vi "TimerHelper.vi"() -> ()   [LabVIEW 2016]
panel:
  in  "Stop":bool
  in  "Pause/Resume":bool
  in  "Start":bool
  in  "Reset":bool
  out "Clock":dbl format="%#_6f"
  # "STOPWATCH"
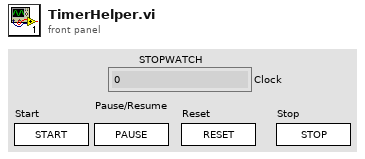
[diagram p1: front panel]
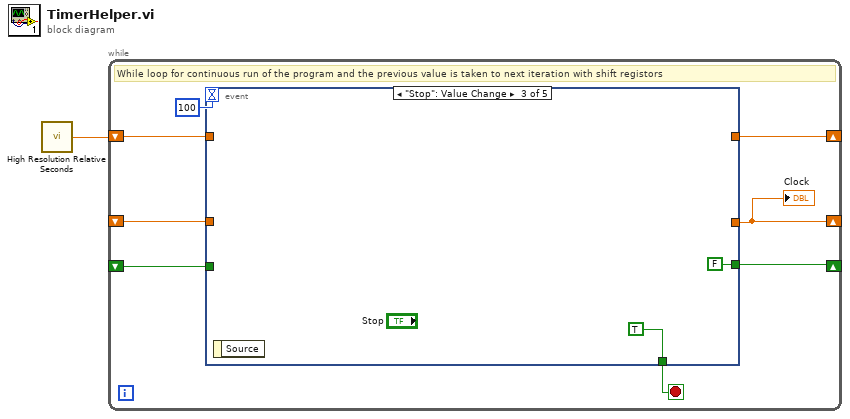
[diagram p0: block diagram]
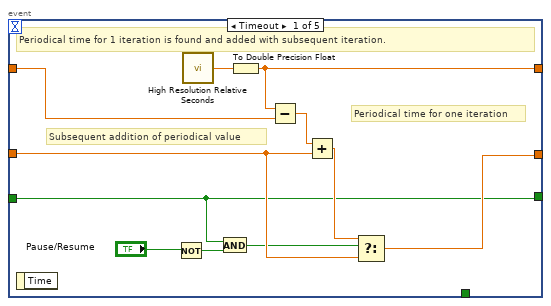
[diagram p2: hidden frame]
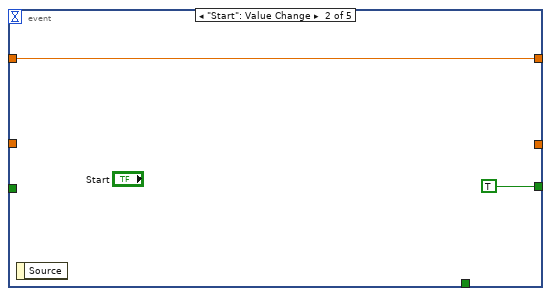
[diagram p3: hidden frame]
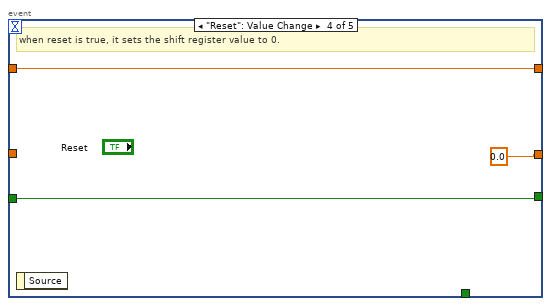
[diagram p4: hidden frame]
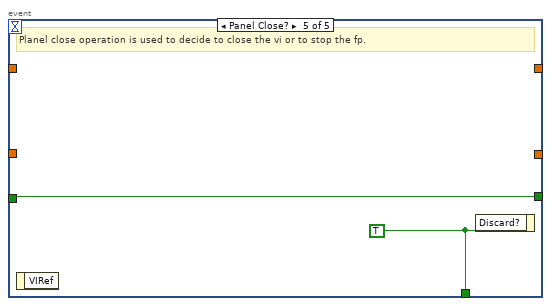
[diagram p5: hidden frame]
diagram:
  n1 = call <vilib>:"High Resolution Relative Seconds.vi"() -> ("relative seconds"=w1:dbl)
  n2 = while {
    shift-right: [w5] -> _
    shift-left: _ -> [w9]
    shift-right: [w8] -> _
    shift-left: w1 -> [w7]
    shift-right: [w3] -> _
    shift-left: _ -> [w2]
    stop <- w4 stop-if-true
    # "While loop for continuous run of the program and the previous value is taken to next iteration with shift registors"
    n3 = event shown="[2] \"Stop\": Value Change" {
      selector: _ -> [_ _ _ _ _]
      dyn-events: _ -> [_ _ _ _ _]
      timeout: 100 -> [_ _ _ _ _]
      tunnel: w9 -> [w20 _ _ _ _]
      tunnel: [w19 w22 _ w27 _] -> w8
      tunnel: [w13 _ _ 0.0 _] -> w5
      tunnel: w7 -> [w18 w22 _ w27 _]
      tunnel: w2 -> [w10 _ _ w25 w28]
      tunnel: [_ _ TRUE _ w29] -> w4
      tunnel: [w10 TRUE FALSE w25 w28] -> w3
      event Timeout {
        # "Subsequent addition of periodical value"
        # "Periodical time for one iteration"
        # "Periodical time for 1 iteration is found and added with subsequent iteration."
        n4 = event-data() -> ()  [unwired: 1 in, 1 out]
        n5 = Not(x="Pause/Resume") -> (.not. x?=w12:bool)
        n6 = call <vilib>:"High Resolution Relative Seconds.vi"() -> ("relative seconds"=w17:dbl)
        n7 = And(x=w10, y=w12) -> (x .and. y?=w11:bool)
        n8 = To Double Precision Float(number=w17) -> (double precision float=w19:dbl)
        n9 = Subtract(x=w19, y=w18) -> (x-y=w15:dbl)
        n10 = Add(x=w15, y=w20) -> (x+y=w16:dbl)
        n11 = Select(t=w16, s=w11, f=w20) -> (s? t:f=w13:dbl)
      }
      event "Start": Value Change {
        n12 = event-data() -> ()  [unwired: 1 in, 1 out]
      }
      event "Stop": Value Change {
        n13 = event-data() -> ()  [unwired: 1 in, 1 out]
      }
      event "Reset": Value Change {
        # "when reset is true, it sets the shift register value to 0."
        n14 = event-data() -> ()  [unwired: 1 in, 1 out]
      }
      event Panel Close? {
        w29 = TRUE
        # "Planel close operation is used to decide to close the vi or to stop the fp."
        n15 = event-data() -> ()  [unwired: 1 in, 1 out]
        n16 = event-data("Discard?"=w29) -> ()  [unwired: 1 in, 1 out]
      }
    }
    "Clock" <- w5
  }
